vi "CSDB_Transfer.get instance data from DB by match pattern.vi"(0 "all instances":string[](array[string]), 2 "match pattern":string, 4 "Data source":string, 5 "error in (no error)":errorcluster) -> (15 "Instances":string[][](array[string]), 17 "data":string[][](array[string]), 19 "error out":errorcluster)   [LabVIEW 2014, in "CSDB_Transfer.lvlib"]
doc: "Reads the data for all instances, which match the pattern, from the DB."
uses:
  CSDB_Transfer.lvlib
  <vilib>/addons/database/Connection.llb/DB Tools Open Connec (String).vi
  <vilib>/addons/database/NI_Database_API.lvlib
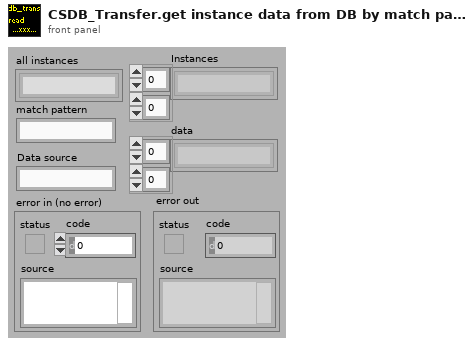
[diagram p1: front panel]
types:
  T1 = typedef "NI_Database_API.lvlib/Conn ObjectReference.ctl" = refnum<k1>
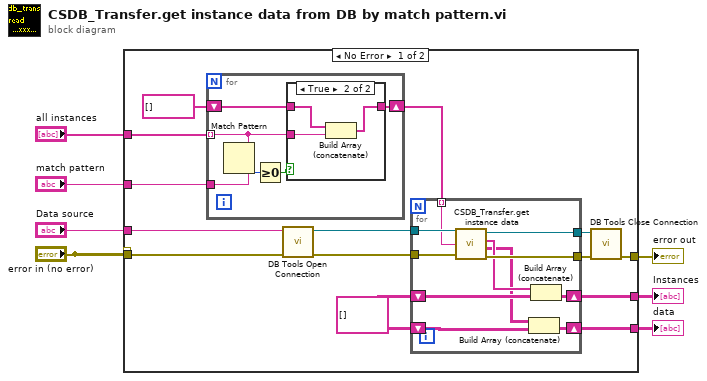
[diagram p0: block diagram]
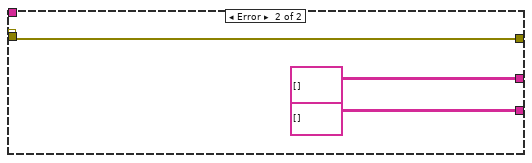
[diagram p3: hidden frame]
diagram:
  n1 = case shown="No Error" "error in (no error)" {
    tunnel: [w14 w45] -> w7
    tunnel: "all instances" -> [w13 _]
    tunnel: "match pattern" -> [w12 _]
    tunnel: "Data source" -> [w11 _]
    tunnel: [w10 string[][] []] -> w3
    tunnel: [w9 string[][] []] -> w2
    tunnel: "error in (no error)" -> [w8 w45]
    frame No Error {
      w17 = string[][] []
      n2 = for {
        tunnel: w13 -> [w37] mode=indexing
        tunnel: w12 -> [w38]
        shift-right: [w35] -> w18
        shift-left: string[] [] -> [w36]
        n3 = Match Pattern(string=w37, regular expression=w38) -> (offset past match=w34:i32)  [unwired: 1 in, 3 out]
        n4 = Greater Or Equal To 0?(x=w34) -> (x >= 0?=w33:bool)
        n5 = case shown="True" w33 {
          tunnel: w37 -> [_ w42]
          tunnel: w36 -> [w39 w41]
          tunnel: [w39 w40] -> w35
          frame False {
          }
          frame True {
            n6 = Build Array (concatenate)(w41, w42) -> (w40:string[])
          }
        }
      }
      n7 = call-poly <vilib>:"DB Tools Open Connection.vi"("error in (no error)"=w8, "connection information"=w11) -> ("error out"=w19:errorcluster, "connection reference"=w20:T1)  [unwired: 6 in]
      n8 = for {
        tunnel: w20 -> [w32]
        tunnel: w19 -> [w31]
        tunnel: w18 -> [w30] mode=indexing
        tunnel: [w29] -> w15
        tunnel: [w28] -> w16
        shift-right: [w25] -> w10
        shift-left: w17 -> [w26]
        shift-right: [w22] -> w9
        shift-left: w17 -> [w23]
        n9 = call "CSDB_Transfer.get instance data.vi"("connection reference"=w32, "InstanceName"=w30, "error in (no error)"=w31) -> ("connection reference out"=w28:T1, "InstanceName      Classname"=w27:string[], "InstanceName      AttributeName      Value"=w24:string[][], "error out"=w29:errorcluster)
        n10 = Build Array (concatenate)(w24, w23) -> (w22:string[][])
        n11 = Build Array (concatenate)(w27, w26) -> (w25:string[][])
      }
      n12 = call <vilib>:"DB Tools Close Connection.vi"("error in (no error)"=w15, "connection reference"=w16) -> ("error out"=w14:errorcluster)  [unwired: 5 in]
    }
    frame Error {
    }
  }
  "error out" <- w7
  "Instances" <- w3
  "data" <- w2
